vi "CVT2ParallelStaticTestNoEr.vi"() -> (3 "Unit Test Framework Results":T1)   [LabVIEW 2012, in "UnitTests.lvlib"]
uses:
  UnitTests.lvlib
  <vilib>/utf/common/utf_test_result_troll.ctl
  <vilib>/utf/common/utf_test_result.ctl
  <vilib>/utf/common/utf_test_result_failure.ctl
  <vilib>/utf/common/utf_test_comparison_operators.ctl
  <vilib>/utf/common/utf_vi_tag.ctl
  CVT3/DataTypes/I32_Static Write.vi
  CVT3/DataTypes/I32_Static Read.vi
  CVT3/Type to Enum.vi
  CVT3/DataTypes/I32_Type To Enum.vi
  CVT3/FGVs/Tag Indices Memory.vi
  CVT3/Errors/Type Mismatch.vi
  CVT3/Memory Block.vi
  CVT3/DataTypes/I32_Memory Block.vi
  <vilib>/utf/NI_UnitTestFramework.lvlib
  CVT3/CVT.lvlib
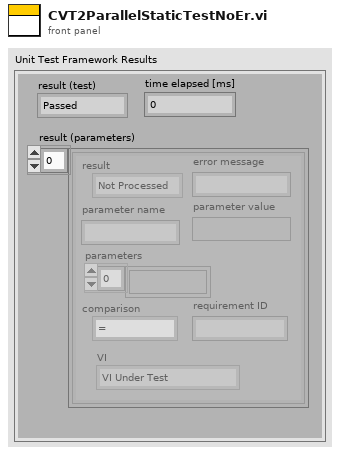
[diagram p1: front panel]
types:
  T1 = typedef "NI_UnitTestFramework.lvlib/utf_test_result_troll.ctl" = cluster{"time elapsed [ms]":u32, "result (test)":T2, "result (parameters)":T3[]}
  T2 = typedef "NI_UnitTestFramework.lvlib/utf_test_result.ctl" = enum16{"Passed", "Failed", "Error", "Skipped", "Not Processed"}
  T3 = typedef "NI_UnitTestFramework.lvlib/utf_test_result_failure.ctl" = cluster{"result":T2, "error message":string, "parameter name":string, "parameter value":variant, "parameters":variant[], "comparison":T4, "requirement ID":string, "VI":T5}
  T4 = typedef "NI_UnitTestFramework.lvlib/utf_test_comparison_operators.ctl" = enum16{"=", "!=", ">", ">=", "<", "<=", "range", "symmetric tolerance", "asymmetric tolerance", "string contains", "string not contain", "array size", "string length", "array range", "by element", "array range (limit array)", "custom", "array contains", "array not contain", "vector length", "= (elm)", "!= (elm)", "= (case insensitive)", "!= (case insensitive)"}
  T5 = typedef "NI_UnitTestFramework.lvlib/utf_vi_tag.ctl" = enum16{"Setup VI", "VI Under Test", "Teardown VI"}
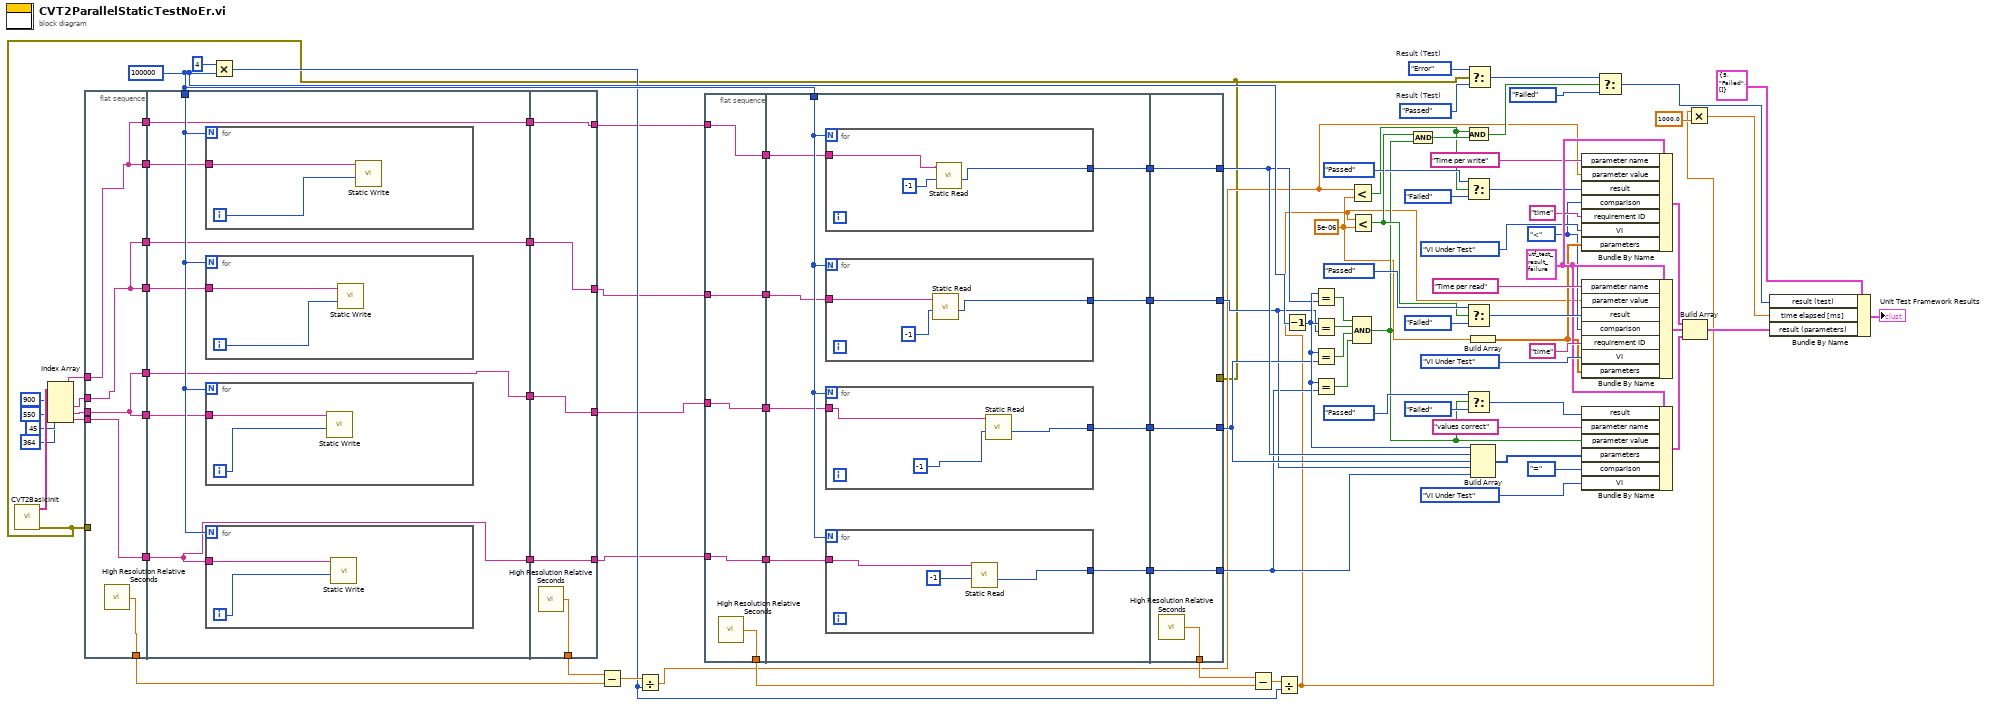
[diagram p0: block diagram]
diagram:
  w52 = T3 {"result"=enum."Passed", "error message"="", "parameter name"="", "parameter value"=variant, "parameters"=[], "comparison"=enum."=", "requirement ID"="", "VI"=enum."Setup VI"} ("Unit Test Framework - result (parameters)")
  w32 = 5e-06 ("y")
  w43 = utf_test_comparison_operators."<" ("comparison")
  w83 = utf_test_result."Error"  # Result (Test)
  w82 = utf_test_result."Passed"  # Result (Test)
  w58 = 100000
  n1 = call "CVT2BasicInit.vi"() -> ("error out"=w1:errorcluster, "names"=w29:string[])  [unwired: 9 in, 1 out]
  n2 = Index Array(array=w29, index #1=900 ("index"), index #2=550 ("index"), index #3=45 ("index"), index #4=364 ("index")) -> (element #1=w18:string, element #2=w19:string, element #3=w21:string, element #4=w24:string)
  n3 = flat-sequence {
    tunnel: [w99] -> w93
    tunnel: w1 -> [_]
    tunnel: w24 -> [w98]
    tunnel: [w98] -> w23
    tunnel: [w95] -> w22
    tunnel: w21 -> [w95]
    tunnel: [w96] -> w20
    tunnel: w19 -> [w96]
    tunnel: w18 -> [w97]
    tunnel: [w97] -> w17
    tunnel: [w97] -> w13
    tunnel: [w96] -> w12
    tunnel: [w95] -> w5
    tunnel: w58 -> [w107]
    tunnel: w23 -> [w100]
    tunnel: w22 -> [w106]
    tunnel: w20 -> [w105]
    tunnel: w17 -> [w104]
    tunnel: [w103] -> w14
    tunnel: w13 -> [w103]
    tunnel: w12 -> [w102]
    tunnel: [w102] -> w11
    tunnel: [w101] -> w6
    tunnel: w5 -> [w101]
    tunnel: [w100] -> w4
    tunnel: [w116] -> w94
    tunnel: [w120] -> w15
    tunnel: w14 -> [w120]
    tunnel: w11 -> [w119]
    tunnel: [w119] -> w10
    tunnel: [w118] -> w7
    tunnel: w6 -> [w118]
    tunnel: w4 -> [w117]
    tunnel: [w117] -> w3
    frame #0 {
      n4 = call <vilib>:"High Resolution Relative Seconds.vi"() -> ("relative seconds"=w99:dbl)
    }
    frame #1 {
      n5 = for {
        N: w107 -> [_]
        tunnel: w104 -> [w115]
        i -> [w114]
        n6 = call-poly "Static Write.vi"("Value"=w114, "Tag Name"=w115) -> ()  [unwired: 9 in, 1 out]
      }
      n7 = for {
        N: w107 -> [_]
        tunnel: w105 -> [w108]
        i -> [w109]
        n8 = call-poly "Static Write.vi"("Value"=w109, "Tag Name"=w108) -> ()  [unwired: 9 in, 1 out]
      }
      n9 = for {
        N: w107 -> [_]
        tunnel: w106 -> [w112]
        i -> [w113]
        n10 = call-poly "Static Write.vi"("Value"=w113, "Tag Name"=w112) -> ()  [unwired: 9 in, 1 out]
      }
      n11 = for {
        N: w107 -> [_]
        tunnel: w100 -> [w111]
        i -> [w110]
        n12 = call-poly "Static Write.vi"("Value"=w110, "Tag Name"=w111) -> ()  [unwired: 9 in, 1 out]
      }
    }
    frame #2 {
      n13 = call <vilib>:"High Resolution Relative Seconds.vi"() -> ("relative seconds"=w116:dbl)
    }
  }
  n14 = Multiply(x=4, y=w58) -> (x*y=w54:i32)
  n15 = Subtract(x=w94, y=w93) -> (x-y=w56:dbl)
  n16 = Divide(x=w56, y=w54) -> (x/y=w30:dbl)
  n17 = flat-sequence {
    tunnel: [w125] -> w92
    tunnel: [w124] -> w16
    tunnel: w15 -> [w124]
    tunnel: w10 -> [w123]
    tunnel: [w123] -> w9
    tunnel: [w122] -> w8
    tunnel: w7 -> [w122]
    tunnel: w3 -> [w121]
    tunnel: [w121] -> w2
    tunnel: [w134] -> w90
    tunnel: [w133] -> w89
    tunnel: [w132] -> w88
    tunnel: [w131] -> w87
    tunnel: w58 -> [w130]
    tunnel: w16 -> [w129]
    tunnel: w9 -> [w128]
    tunnel: w8 -> [w127]
    tunnel: w2 -> [w126]
    tunnel: [w151] -> w91
    tunnel: w90 -> [w150]
    tunnel: w89 -> [w149]
    tunnel: w88 -> [w148]
    tunnel: w87 -> [w147]
    tunnel: w1 -> [_]
    tunnel: [w150] -> w36
    tunnel: [w149] -> w34
    tunnel: [w148] -> w35
    tunnel: [w147] -> w33
    frame #0 {
      n18 = call <vilib>:"High Resolution Relative Seconds.vi"() -> ("relative seconds"=w125:dbl)
    }
    frame #1 {
      n19 = for {
        N: w130 -> [_]
        tunnel: [w146] -> w134
        tunnel: w129 -> [w145]
        n20 = call-poly "Static Read.vi"("Default"=-1, "Tag Name"=w145) -> ("Value"=w146:i32)  [unwired: 8 in, 1 out]
      }
      n21 = for {
        N: w130 -> [_]
        tunnel: [w135] -> w133
        tunnel: w128 -> [w137]
        n22 = call-poly "Static Read.vi"("Default"=-1, "Tag Name"=w137) -> ("Value"=w135:i32)  [unwired: 8 in, 1 out]
      }
      n23 = for {
        N: w130 -> [_]
        tunnel: [w143] -> w132
        tunnel: w127 -> [w141]
        n24 = call-poly "Static Read.vi"("Default"=-1, "Tag Name"=w141) -> ("Value"=w143:i32)  [unwired: 8 in, 1 out]
      }
      n25 = for {
        N: w130 -> [_]
        tunnel: [w138] -> w131
        tunnel: w126 -> [w139]
        n26 = call-poly "Static Read.vi"("Default"=-1, "Tag Name"=w139) -> ("Value"=w138:i32)  [unwired: 8 in, 1 out]
      }
    }
    frame #2 {
      n27 = call <vilib>:"High Resolution Relative Seconds.vi"() -> ("relative seconds"=w151:dbl)
    }
  }
  n28 = Subtract(x=w91, y=w92) -> (x-y=w55:dbl)
  n29 = Divide(x=w55, y=w54) -> (x/y=w31:dbl)
  n30 = Decrement(x=w58) -> (x-1=w37:i32)
  n31 = Equal?(x=w37, y=w36) -> (x = y?=w59:bool)
  n32 = Equal?(x=w37, y=w34) -> (x = y?=w60:bool)
  n33 = Equal?(x=w37, y=w35) -> (x = y?=w61:bool)
  n34 = Equal?(x=w37, y=w33) -> (x = y?=w62:bool)
  n35 = Less?(x=w30, y=w32) -> (x < y?=w39:bool)
  n36 = Less?(x=w31, y=w32) -> (x < y?=w70:bool)
  n37 = Compound Arithmetic op=AND(w59, w60, w61, w62) -> (w38:bool)
  n38 = And(x=w70, y=w38) -> (x .and. y?=w48:bool)
  n39 = And(x=w39, y=w48) -> (x .and. y?=w47:bool)
  n40 = Select(t=utf_test_result."Passed" ("result"), s=w39, f=utf_test_result."Failed" ("result")) -> (s? t:f=w40:T2)
  n41 = Select(t=utf_test_result."Passed" ("result"), s=w70, f=utf_test_result."Failed" ("result")) -> (s? t:f=w73:T2)
  n42 = Select(t=utf_test_result."Passed" ("result"), s=w38, f=utf_test_result."Failed" ("result")) -> (s? t:f=w66:T2)
  n43 = Select(t=w83, s=w1, f=w82) -> (s? t:f=w78:T2)
  n44 = Build Array(w32) -> (w44:dbl[])
  n45 = Build Array(w37, w36, w35, w34, w33) -> (w64:i32[])
  n46 = Bundle By Name(cluster=w52, "parameter name"="Time per write", "parameter value"=w30, "result"=w40, "comparison"=w43, "requirement ID"="time", "VI"=utf_vi_tag."VI Under Test", "parameters"=w44) -> (w53:T3)
  n47 = Bundle By Name(cluster=w52, "parameter name"="Time per read", "parameter value"=w31, "result"=w73, "comparison"=w43, "requirement ID"="time", "VI"=utf_vi_tag."VI Under Test", "parameters"=w44) -> (w51:T3)
  n48 = Bundle By Name(cluster=w52, "result"=w66, "parameter name"="values correct", "parameter value"=w38, "parameters"=w64, "comparison"=utf_test_comparison_operators."=", "VI"=utf_vi_tag."VI Under Test") -> (w50:T3)
  n49 = Select(t=w78, s=w47, f=utf_test_result."Failed") -> (s? t:f=w76:T2)
  n50 = Build Array(w53, w51, w50) -> (w81:T3[])
  n51 = Multiply(x=w31, y=1000.0) -> (x*y=w79:dbl)
  n52 = Bundle By Name(cluster=T1 {"time elapsed [ms]"=5, "result (test)"=enum."Failed", "result (parameters)"=[]} ("Unit Test Framework - Result"), "result (test)"=w76, "time elapsed [ms]"=w79, "result (parameters)"=w81) -> (→"Unit Test Framework Results":T1)
